vi "BC Wrapper.vi"(0 "File To Program":path, 2 "Console Ref":refnum<vi>, 7 "BootCommander Folder":path, 11 "Error In":errorcluster) -> (4 "StdOut":string, 6 "Std Error":string, 15 "error out":errorcluster)   [LabVIEW 2021]
doc: "It's wrapper for the BootCommander.exe"
uses:
  <vilib>/JKI/JKI DotNet System Exec/dotnet_system_exec/dotnet_system_exec.lvclass
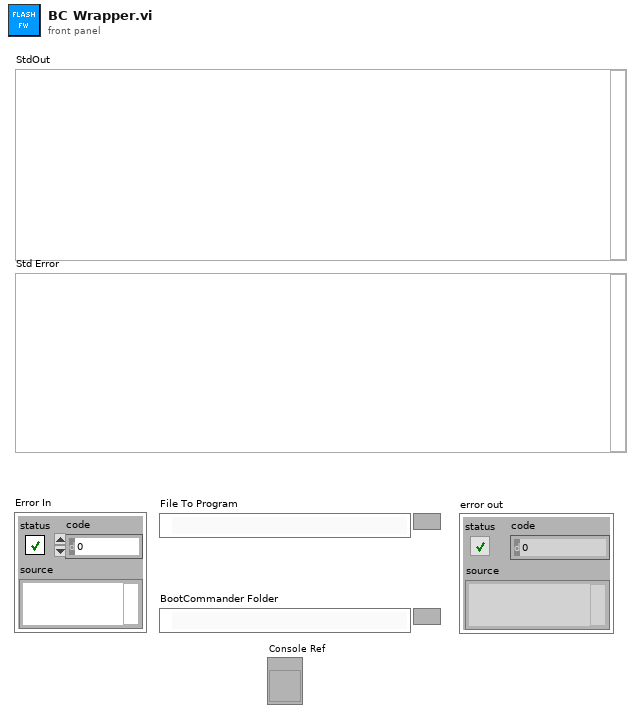
[diagram p1: front panel]
types:
  T1 = cluster{"stdout event":refnum<user-event>, "stderr event":refnum<user-event>, "process_exit event":refnum<user-event>}
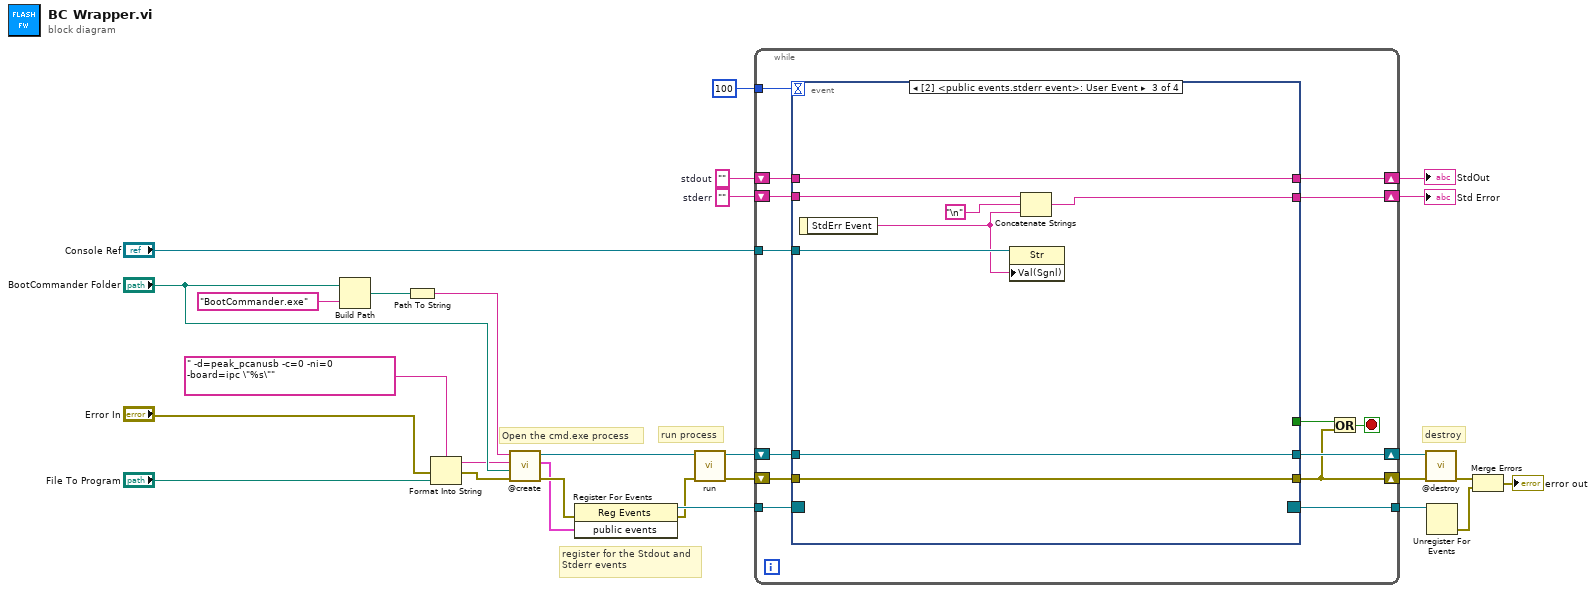
[diagram p0: block diagram]
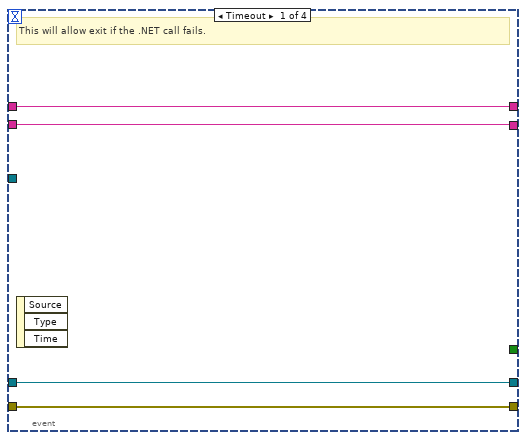
[diagram p2: hidden frame]
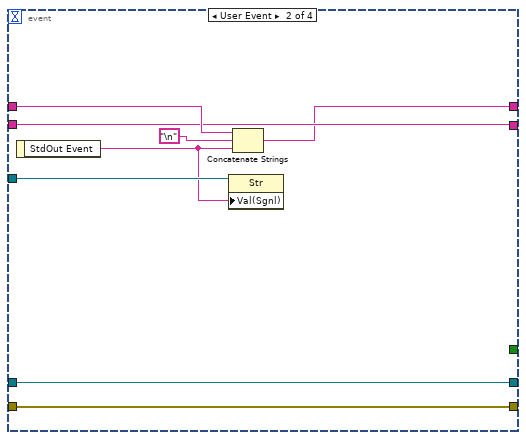
[diagram p3: hidden frame]
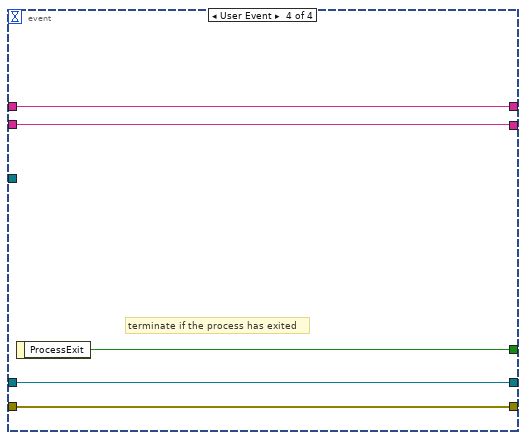
[diagram p4: hidden frame]
diagram:
  w17 = ""  # stderr
  w21 = ""  # stdout
  # "destroy"
  # "register for the Stdout and\nStderr events"
  # "run process"
  # "Open the cmd.exe process"
  n1 = Build Path(base path="BootCommander Folder", name or relative path="BootCommander.exe") -> (appended path=w10:path)
  n2 = Path To String(path=w10) -> (string=w9:string)
  n3 = Format Into String(format string=" -d=peak_pcanusb -c=0 -ni=0 -board=ipc \"%s\"" ("string"), error in="Error In", "File To Program") -> (resulting string=w6:string, error out=w7:errorcluster)  [unwired: 1 in]
  n4 = call <vilib>:"@create.vi"("error in (no error)"=w7, "working directory (c:\\)"="BootCommander Folder", "arguments (\"\")"=w6, "command line (cmd.exe)"=w9) -> ("error out"=w20:errorcluster, "public events"=w18:T1, "dotnet_system_exec out"=w27:refnum<class "dotnet_system_exec.lvclass">)  [unwired: 5 in]
  n5 = register-events(error in=w20, w18) -> (reference out=w26:refnum<event-registration>, error out=w19:errorcluster)  [unwired: 1 in]
  n6 = call <vilib>:"run.vi"("error in (no error)"=w19, "dotnet_system_exec in"=w27) -> ("error out"=w15:errorcluster, "dotnet_system_exec out"=w16:refnum<class "dotnet_system_exec.lvclass">)  [unwired: 8 in]
  n7 = while {
    shift-right: [w42] -> w28
    shift-left: w16 -> [w41]
    shift-right: [w31] -> w24
    shift-left: w15 -> [w40]
    tunnel: w26 -> [w39]
    tunnel: [w38] -> w25
    shift-right: [w36] -> w2
    shift-left: w21 -> [w37]
    shift-right: [w34] -> w1
    shift-left: w17 -> [w35]
    tunnel: 100 -> [w30]
    tunnel: "Console Ref" -> [w29]
    stop <- w33 stop-if-true
    n8 = event shown="[2] <public events.stderr event>: User Event" {
      selector: w39 -> [_ _ _ _]
      dyn-events: [_ _ _ _] -> w38
      timeout: w30 -> [_ _ _ _]
      tunnel: [w46 w54 w62 w64] -> w42
      tunnel: w41 -> [w46 w54 w62 w64]
      tunnel: w40 -> [w45 w50 w61 w63]
      tunnel: [w45 w50 w61 w63] -> w31
      tunnel: w37 -> [w44 w52 w58 w65]
      tunnel: [w44 w49 w58 w65] -> w36
      tunnel: [_ _ _ w67] -> w32
      tunnel: w35 -> [w43 w51 w59 w66]
      tunnel: [w43 w51 w57 w66] -> w34
      tunnel: w29 -> [_ w48 w56 _]
      event Timeout {
        # "This will allow exit if the .NET call fails."
        n9 = event-data() -> ()  [unwired: 1 in, 3 out]
      }
      event User Event {
        n10 = event-data() -> ("StdOut Event"=w47:string)  [unwired: 1 in]
        n11 = property class="Str"(reference=w48, "Val(Sgnl)"=w47) -> ()  [unwired: 1 in, 2 out]
        n12 = Concatenate Strings(w52, "\n", w47) -> (w49:string)
      }
      event User Event {
        n13 = event-data() -> ("StdErr Event"=w55:string)  [unwired: 1 in]
        n14 = property class="Str"(reference=w56, "Val(Sgnl)"=w55) -> ()  [unwired: 1 in, 2 out]
        n15 = Concatenate Strings(w59, "\n", w55) -> (w57:string)
      }
      event User Event {
        # "terminate if the process has exited"
        n16 = event-data() -> ("ProcessExit"=w67:bool)  [unwired: 1 in]
      }
    }
    n17 = Or(x=w32, y=w31) -> (x .or. y?=w33:bool)
  }
  "StdOut" <- w2
  "Std Error" <- w1
  n18 = call-dynamic "@destroy.vi"("error in (no error)"=w24, "dotnet_system_exec in"=w28) -> ("error out"=w23:errorcluster)  [unwired: 8 in, 1 out]
  n19 = Unregister For Events(event registration refnum=w25) -> (error out=w22:errorcluster)  [unwired: 1 in]
  n20 = Merge Errors(w23, w22) -> (→"error out":errorcluster)
